vi "Barcode read.vi"(8 "error in":errorcluster, 11 "queue in":refnum<queue>) -> (0 "error out":errorcluster, 1 "exit":bool, 2 "read buffer":string, 3 "queue Out 2":refnum<queue>)   [LabVIEW 2020]
uses:
  Test  enqueue/AutoTest seq.ctl
  <vilib>/Instr/_visa.llb/VISA Configure Serial Port (Instr).vi
  Galobal variable_TI.vi
  Project Setup/Globle Variable/GR_Servo.vi
panel:
  out "x = y?":bool
  out "substring":string
  out "error out 2":errorcluster
  out "error out":errorcluster
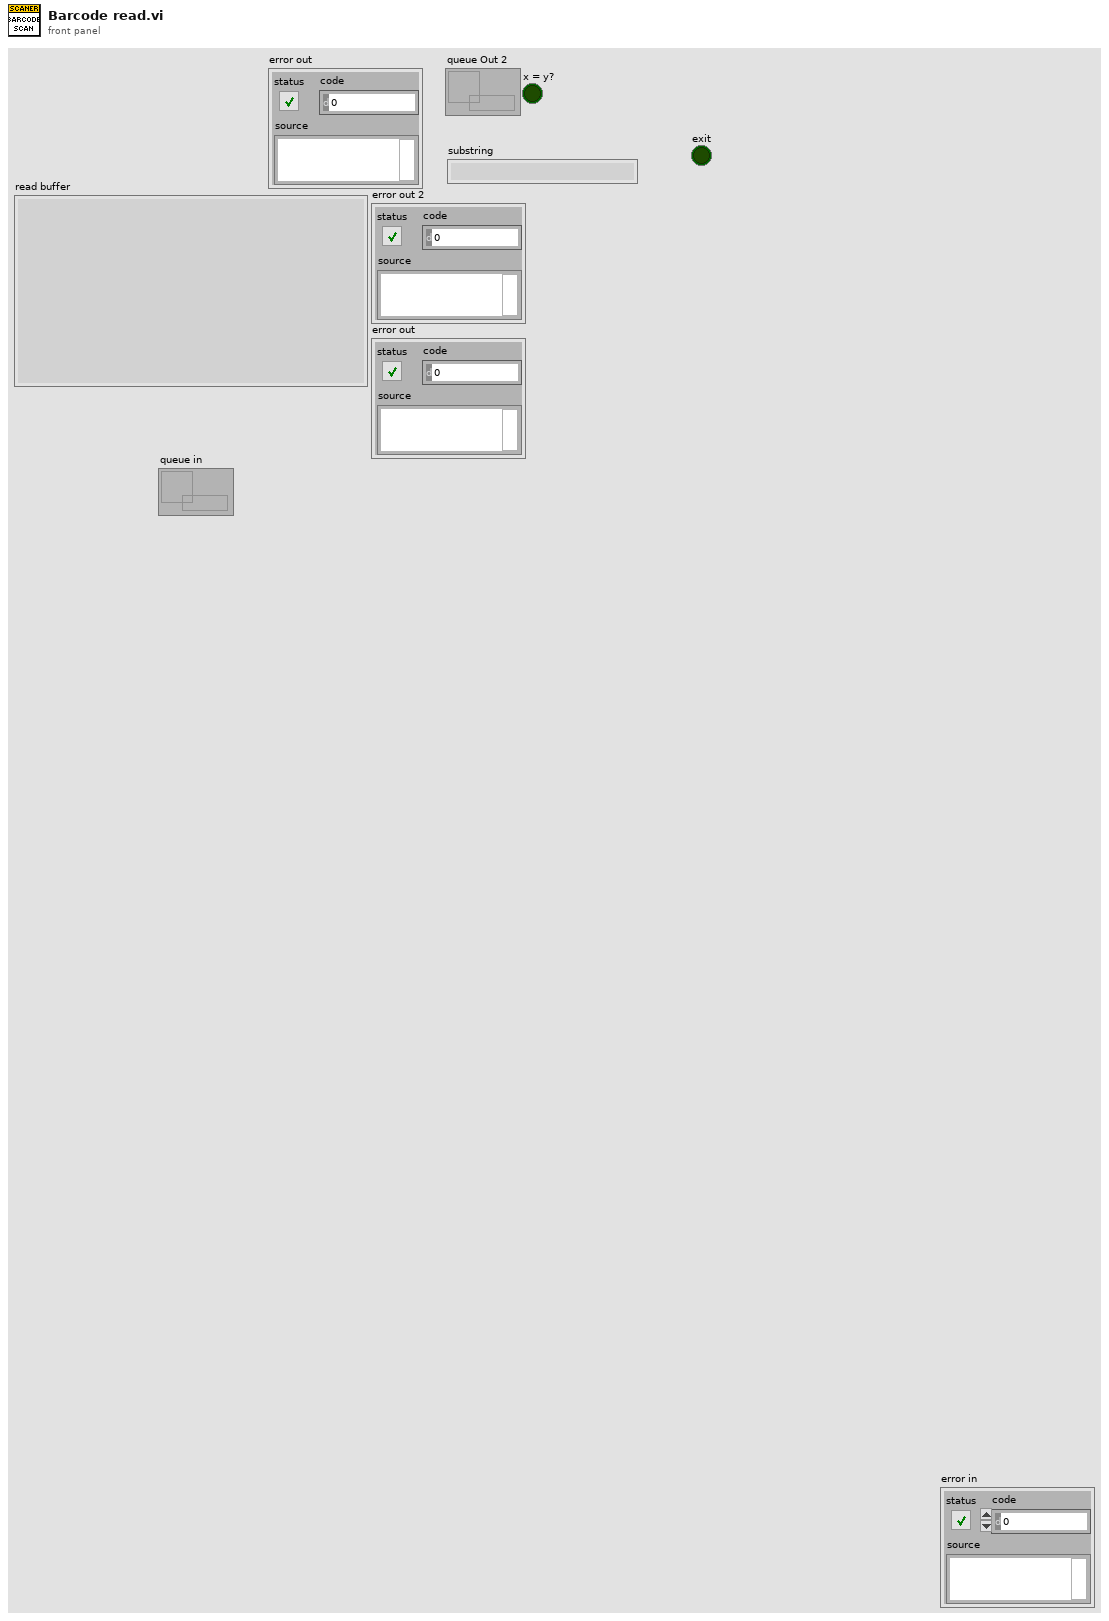
[diagram p1: front panel]
types:
  T1 = cluster{"MaxLoad ":dbl, "Min Load":dbl, "MaxDistance(mm)":dbl, "Min Distance(mm)":dbl, "Load Offset":dbl, "Model":string, "Difusser Code":string, "TFT Code ":string, "LVDT Offset":dbl}
  T2 = cluster{"Start":bool, "Emergency ":bool, "Reset":bool, "Home":bool, "Safety":bool}
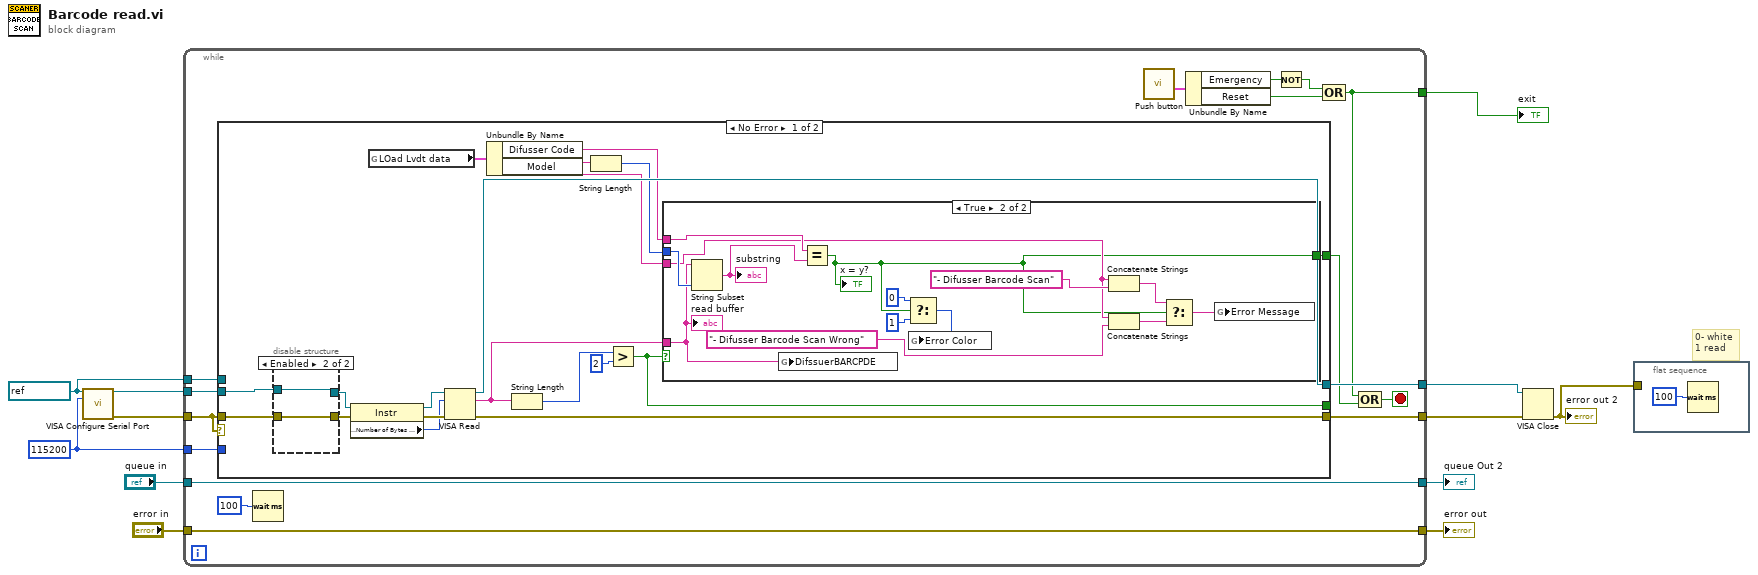
[diagram p0: block diagram]
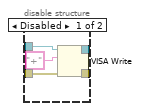
[diagram p2: hidden frame]
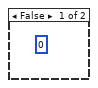
[diagram p3: hidden frame]
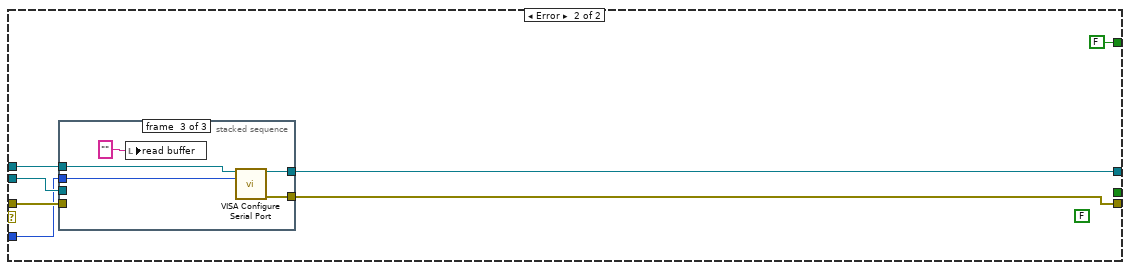
[diagram p4: hidden frame]
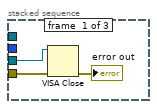
[diagram p5: hidden frame]
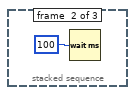
[diagram p6: hidden frame]
diagram:
  w7 = u32 115200 ("baud rate (9600)")
  w8 = refnum<visa-resource-name> "COM1" ("VISA resource name")
  # "0- white\n1 read"
  n1 = call-poly "VISA Configure Serial Port"("VISA resource name"=w8, "baud rate (9600)"=w7) -> ("VISA resource name out"=w12:refnum<visa-resource-name>, "error out"=w11:errorcluster)  [unwired: 12 in]
  n2 = while {
    tunnel: w12 -> [w28]
    tunnel: w11 -> [w26]
    tunnel: [w15] -> w10
    tunnel: [w27] -> w9
    tunnel: w8 -> [w25]
    tunnel: w7 -> [w24]
    tunnel: [w13] -> w6
    tunnel: [w21] -> w4
    tunnel: "queue in" -> [w21]
    tunnel: "error in" -> [w20]
    tunnel: [w20] -> w2
    stop <- w22 stop-if-true
    n3 = case shown="No Error" w26 {
      tunnel: w28 -> [w46 w74]
      tunnel: w26 -> [w45 w73]
      tunnel: [w44 w70] -> w15
      tunnel: [w43 w69] -> w27
      tunnel: w25 -> [_ w72]
      tunnel: w24 -> [_ w71]
      tunnel: [w30 FALSE] -> w14
      tunnel: [w29 _] -> _
      frame No Error {
        n4 = disable-structure shown="Enabled" {
          disable-tunnel: w46 -> [w51 w53]
          disable-tunnel: w45 -> [w50 w52]
          disable-tunnel: [w49 w52] -> w42
          disable-tunnel: [w48 w53] -> w41
          frame Disabled {
            n5 = VISA Write(VISA resource name=w51, write buffer="+", error in (no error)=w50) -> (VISA resource name out=w48:refnum<visa-resource-name>, error out=w49:errorcluster)  [unwired: 1 out]
          }
          frame Enabled {
          }
        }
        n6 = property class="Instr"(reference=w41, error in=w42) -> (reference out=w40:refnum<visa-resource-name>, error out=w39:errorcluster, "Serial Settings:Number of Bytes at Serial Port"=w38:u32)
        n7 = global read "Galobal variable_TI.vi" "LOad Lvdt data"() -> (w34:T1)
        n8 = VISA Read(VISA resource name=w40, byte count=w38, error in (no error)=w39) -> (VISA resource name out=w44:refnum<visa-resource-name>, read buffer=w35:string, error out=w43:errorcluster)  [unwired: 1 out]
        n9 = Unbundle By Name(w34) -> ("Difusser Code"=w33:string, "Model"=w31:string)
        n10 = String Length(string=w35) -> (length=w37:i32)
        n11 = String Length(string=w33) -> (length=w32:i32)
        n12 = Greater?(x=w37, y=2) -> (0:w29:bool)
        n13 = case shown="True" w29 {
          tunnel: w35 -> [_ w61]
          tunnel: w33 -> [_ w66]
          tunnel: w32 -> [_ w67]
          tunnel: w31 -> [_ w56]
          tunnel: [_ w54] -> w30
          frame False {
            (unwired) 0 ("f")
          }
          frame True {
            n14 = String Subset(string=w61, length (rest)=w67) -> (substring=w65:string)  [unwired: 1 in]
            "substring" <- w65
            n15 = global write "Galobal variable_TI.vi" "DifssuerBARCPDE"(w61) -> ()
            n16 = Equal?(x=w66, y=w65) -> (x = y?=w54:bool)
            "x = y?" <- w54
            n17 = Select(t=0, s=w54, f=1) -> (s? t:f=w62:i32)
            n18 = global write "GR_Servo.vi" "Error Color"(w62) -> ()
            n19 = Concatenate Strings(w56, "- Difusser Barcode Scan" ("string")) -> (w59:string)
            n20 = Concatenate Strings(w56, "- Difusser Barcode Scan Wrong" ("string")) -> (w58:string)
            n21 = Select(t=w59, s=w54, f=w58) -> (s? t:f=w57:string)
            n22 = global write "GR_Servo.vi" "Error Message"(w57) -> ()
            "read buffer" <- w61
          }
        }
      }
      frame Error {
        (unwired) FALSE
        n23 = stacked-sequence {
          tunnel: w74 -> [w76 _ _]
          tunnel: w73 -> [w75 _ _]
          tunnel: w72 -> [_ _ w83]
          tunnel: w71 -> [_ _ w82]
          tunnel: [_ _ w81] -> w70
          tunnel: [_ _ w80] -> w69
          frame #0 {
            n24 = VISA Close(VISA resource name=w76, error in (no error)=w75) -> (error out=→"error out":errorcluster)
          }
          frame #1 {
            n25 = Wait (ms)(milliseconds to wait=u32 100) -> ()  [unwired: 1 out]
          }
          frame #2 {
            n26 = local write "read buffer"("" ("read buffer")) -> ()
            n27 = call-poly "VISA Configure Serial Port"("VISA resource name"=w83, "baud rate (9600)"=w82) -> ("VISA resource name out"=w81:refnum<visa-resource-name>, "error out"=w80:errorcluster)  [unwired: 12 in]
          }
        }
      }
    }
    n28 = Wait (ms)(milliseconds to wait=u32 100) -> ()  [unwired: 1 out]
    n29 = call "Push button.vi"() -> ("Push Button"=w19:T2)  [unwired: 11 in]
    n30 = Unbundle By Name(w19) -> ("Emergency"=w18:bool, "Reset"=w16:bool)
    n31 = Not(x=w18) -> (.not. x?=w17:bool)
    n32 = Compound Arithmetic op=OR(w17, w16) -> (w13:bool)
    n33 = Compound Arithmetic op=OR(w13, w14) -> (w22:bool)
  }
  "exit" <- w6
  "queue Out 2" <- w4
  "error out" <- w2
  n34 = VISA Close(VISA resource name=w10, error in (no error)=w9) -> (error out=w1:errorcluster)
  "error out 2" <- w1
  n35 = flat-sequence {
    tunnel: w1 -> [_]
    frame #0 {
      n36 = Wait (ms)(milliseconds to wait=u32 100) -> ()  [unwired: 1 out]
    }
  }
